vi "Sort Fcurve wfms_V1.vi"(0 "reference in":refnum<class "Fcurve.lvclass">, 1 "Channels In":waveform(dbl)[](array[waveform]), 5 "error in (no error)":errorcluster) -> (7 "Fcurve out":cluster{"X":dbl[], "Y":dbl[]}[](graph), 14 "reference out":refnum<class "Fcurve.lvclass">, 19 "error out":errorcluster)   [LabVIEW 2019, in "Fcurve.lvclass"]
doc: "Sorts wfms into Fcurve. [0] Deflection, [1] Zposition"
uses:
  Fcurve.lvclass
  Zero Type.ctl
  TDMS_DataHandler_class/property name combo box.ctl
  TDMS_DataHandler_class/TDMS_DataHandler.lvclass
panel:
  in  "Zero type":T1
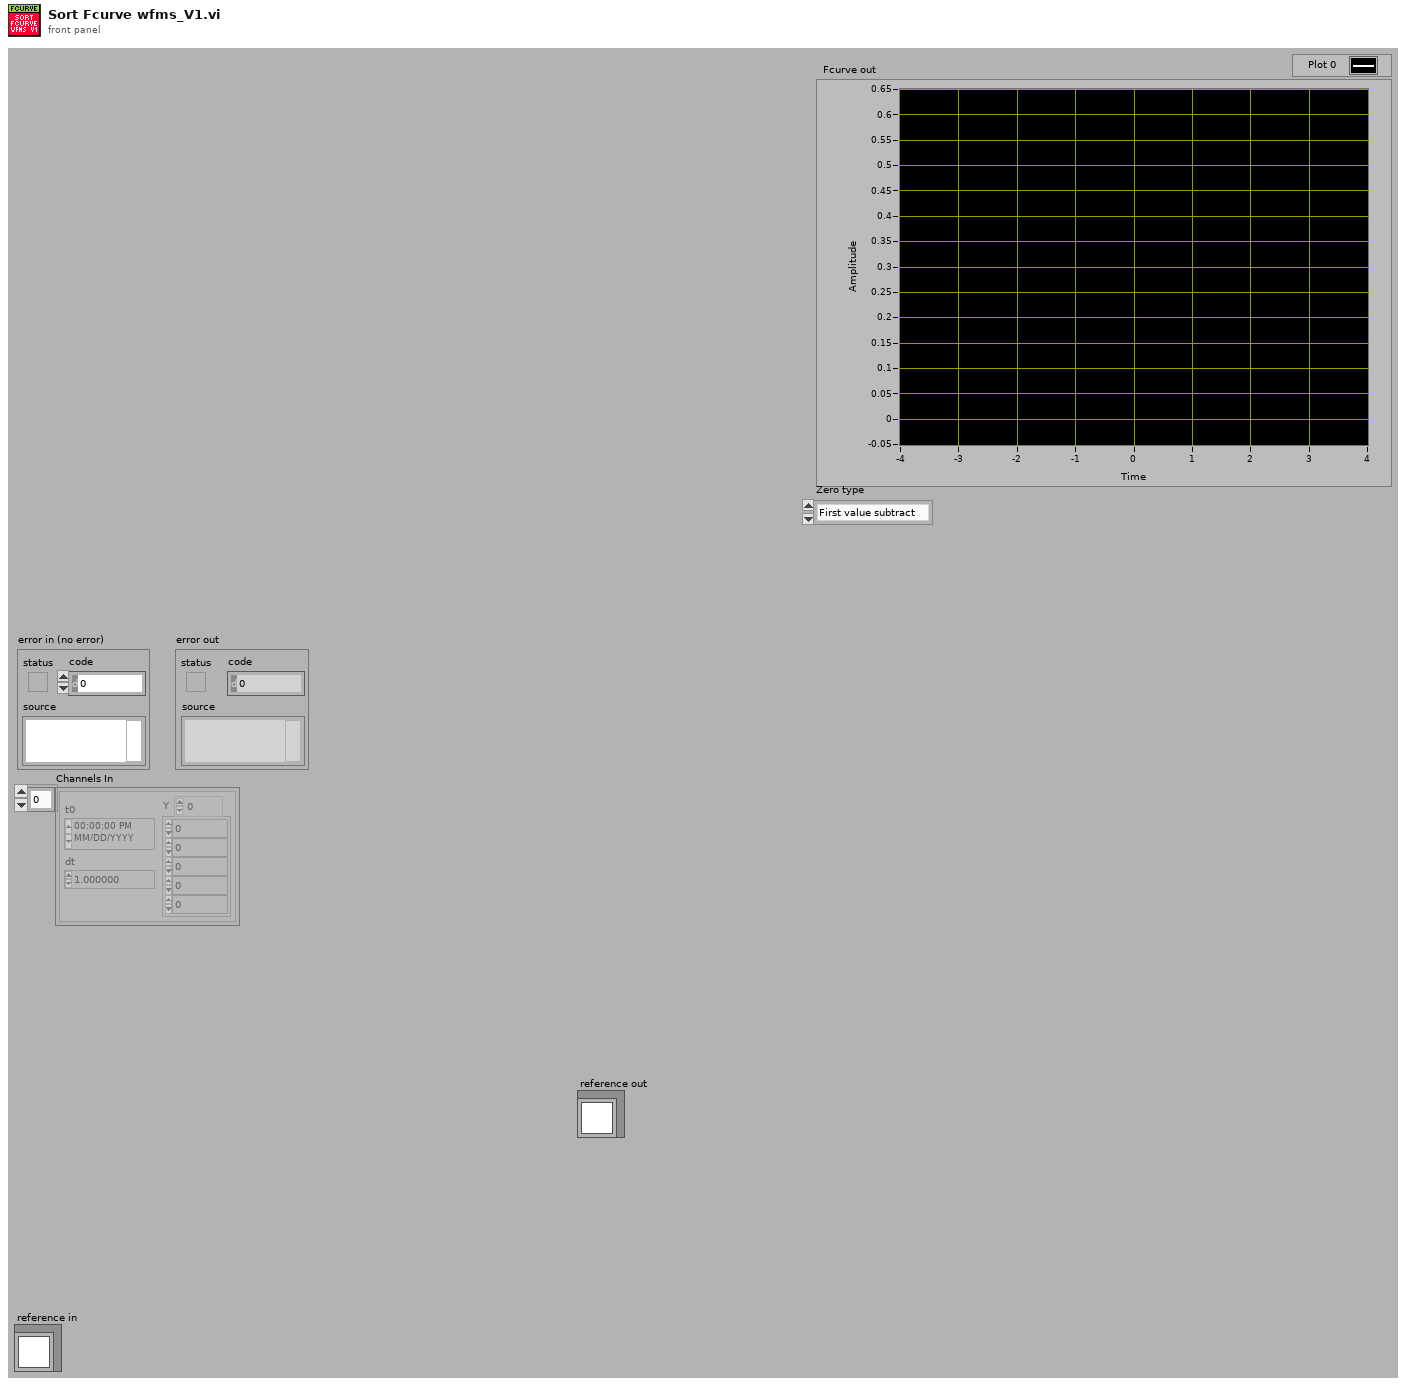
[diagram p1: front panel]
types:
  T1 = typedef "Fcurve.lvclass/Zero Type.ctl" = enum16{"First value subtract", "Median (approach)", "Linear fit (approach)"}
  T2 = typedef "TDMS_DataHandler.lvclass/property name combo box.ctl" = string
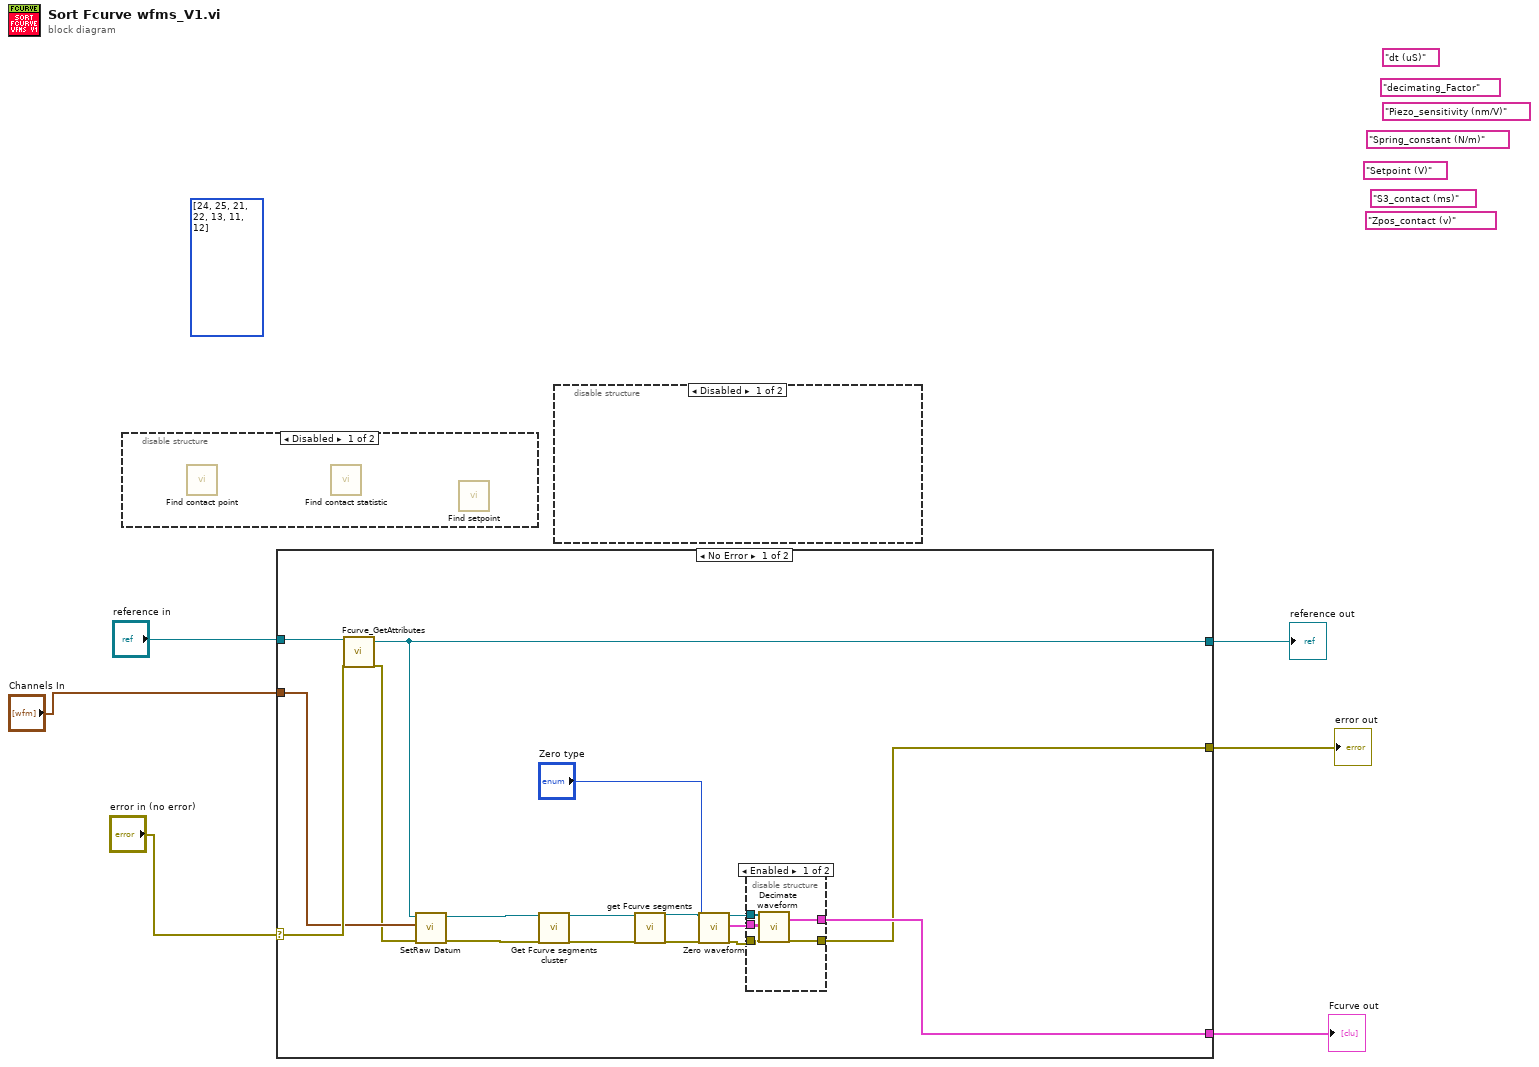
[diagram p0: block diagram]
diagram:
  (unwired) i32[] [24, 25, 21, 22, 13, 11, 12] ("Array")
  (unwired) T2 "Setpoint (V)" ("Combo Box")
  (unwired) T2 "S3_contact (ms)" ("Combo Box")
  (unwired) T2 "Zpos_contact (v)" ("Combo Box")
  (unwired) T2 "Spring_constant (N/m)" ("Combo Box")
  (unwired) T2 "Piezo_sensitivity (nm/V)" ("Combo Box")
  (unwired) T2 "decimating_Factor" ("Combo Box")
  (unwired) T2 "dt (uS)" ("Combo Box")
  n1 = disable-structure shown="Disabled" {
    frame Disabled {
      n2 = call "Find contact point.vi"() -> ()  [unwired: 17 in, 3 out]
      n3 = call "Find contact statistic.vi"() -> ()  [unwired: 17 in, 3 out]
      n4 = call "Find setpoint.vi"() -> ()  [unwired: 17 in, 3 out]
    }
    frame Enabled {
    }
  }
  n5 = case shown="No Error" "error in (no error)" {
    selector: "error in (no error)" -> [w22 w31]
    tunnel: "reference in" -> [w23 w32]
    tunnel: [w17 w32] -> w5
    tunnel: [w20 w31] -> w4
    tunnel: [w21 _] -> w2
    tunnel: "Channels In" -> [w19 _]
    frame No Error {
      n6 = call "Fcurve_GetAttributes.vi"("reference in"=w23, "error in (no error)"=w22) -> ("reference out"=w17:refnum<class "Fcurve.lvclass">, "error out"=w18:errorcluster)  [unwired: 14 in, 2 out]
      n7 = call-dynamic "SetRaw Datum.vi"("error in (no error)"=w18, "Raw Datum"=w19, "reference in"=w17) -> ("error out"=w15:errorcluster, "reference out"=w16:refnum<class "Fcurve.lvclass">)  [unwired: 7 in]
      n8 = call-dynamic "Get Fcurve segments cluster.vi"("reference in"=w16, "error in (no error)"=w15) -> ("reference out"=w13:refnum<class "Fcurve.lvclass">, "error out"=w14:errorcluster)  [unwired: 16 in]
      n9 = call-dynamic "get Fcurve segments.vi"("reference in"=w13, "error in (no error)"=w14) -> ("reference out"=w12:refnum<class "Fcurve.lvclass">, "error out"=w10:errorcluster)  [unwired: 15 in, 1 out]
      n10 = call-dynamic "Zero waveform.vi"("reference in"=w12, "Zero type"="Zero type", "error in (no error)"=w10) -> ("reference out"=w11:refnum<class "Fcurve.lvclass">, "Zero Fcurve Segments"=w8:cluster{"X":dbl[], "Y":dbl[]}[], "error out"=w9:errorcluster)  [unwired: 12 in, 2 out]
      n11 = disable-structure shown="Enabled" {
        disable-tunnel: [w28 w30] -> w21
        disable-tunnel: [w27 w29] -> w20
        disable-tunnel: w11 -> [w26 _]
        disable-tunnel: w9 -> [w25 w29]
        disable-tunnel: w8 -> [w24 w30]
        frame Enabled {
          n12 = call-dynamic "Decimate waveform.vi"("reference in"=w26, "Segment zeroed fcurve data"=w24, "error in (no error)"=w25) -> ("Decimated Fcurve (App,Con,Ret)"=w28:cluster{"X":dbl[], "Y":dbl[]}[], "error out"=w27:errorcluster)  [unwired: 14 in, 1 out]
        }
        frame Disabled {
        }
      }
    }
    frame Error {
    }
  }
  "error out" <- w4
  "reference out" <- w5
  "Fcurve out" <- w2
  n13 = disable-structure shown="Disabled" {
    frame Disabled {
    }
    frame Enabled {
    }
  }
